vi "ReadBlueSerializableVersionPath.vi"(10 "apprefnum":u32, 11 "LVClass name":string) -> (0 "error out":errorcluster, 2 "BlueSerializableVersion found?":bool, 3 "BlueSerializableVersion":u16)   [LabVIEW 2019, in "IncrementMutationHistory.lvlib"]
uses:
  IncrementMutationHistory.lvlib
  <resource>/Framework/Providers/BlueSerializationProviderShared/UserCommentToVersion.vi
  <resource>/Framework/Providers/BlueSerializationProviderShared/BlueSerializationProviderShared.lvlib
  VILIB_NONUI/VILIB_NONUI.lvlib
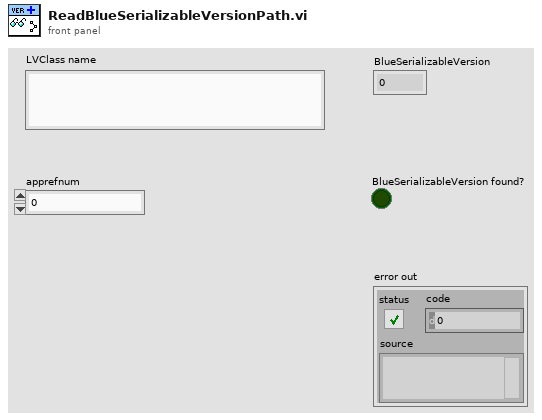
[diagram p1: front panel]
types:
  T1 = typedef "Edit LVLibs.lvlib/Mutation History.ctl" = T2[]
  T2 = typedef "Edit LVLibs.lvlib/Mutation Record.ctl" = cluster{"Library Version":T3, "Old Name Index":u8, "Class Default Data":variant, "Cluster Order Map":u32[], "Parent Name":string, "Parent Path":path, "LabVIEW Version":u32, "User Comments":string, "Mutation Flags":u8, "Parent Old Name Index":u8, "Parent Levels Added":u16, "Parent Levels Removed":u16}
  T3 = typedef "Edit LVLibs.lvlib/LibVersion.ctl" = cluster{"Major":u16, "Minor":u16, "Fix":u16, "Build":u16}
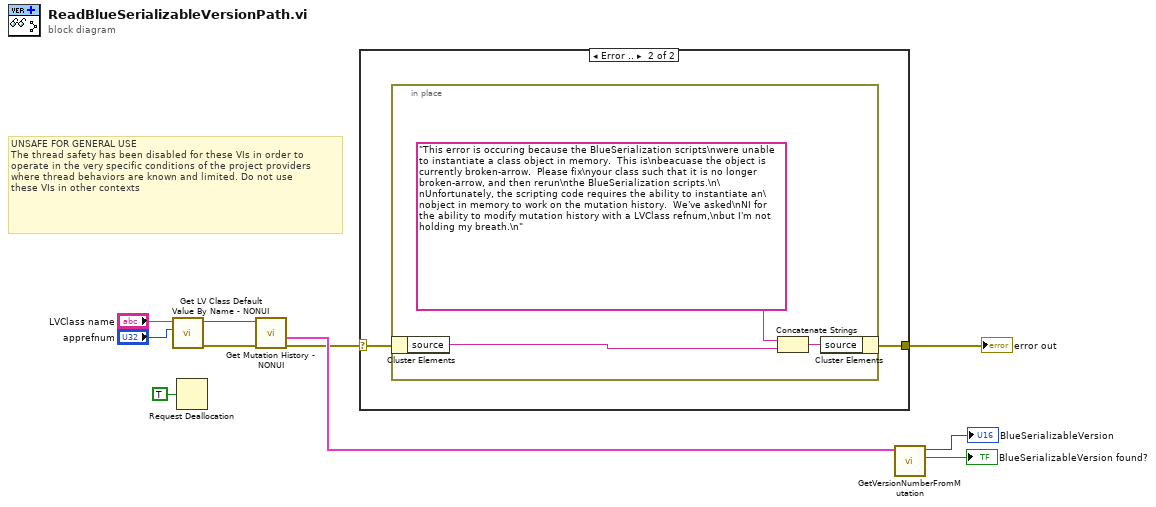
[diagram p0: block diagram]
diagram:
  # "UNSAFE FOR GENERAL USE\nThe thread safety has been disabled for these VIs in order to\noperate in the very specific conditions of the project providers\nwhere thread behaviors are known and limited. Do not use\nthese VIs in other contexts"
  n1 = call "Get LV Class Default Value By Name - NONUI.vi"("apprefnum"="apprefnum", "class name"="LVClass name") -> ("error out"=w5:errorcluster, "object"=w6:refnum<class>)  [unwired: 8 in]
  n2 = Request Deallocation(TRUE ("flag")) -> ()
  n3 = call "Get Mutation History - NONUI.vi"("error in"=w5, "Input object"=w6) -> ("error out"=w2:errorcluster, "Mutation History"=w4:T1)  [unwired: 6 in]
  n4 = case shown="Error .." w2 {
    selector: w2 -> [w11 w13]
    tunnel: [w11 w12] -> w1
    frame No Error {
    }
    frame Error {
      n5 = in-place {
        n6 = in-place-cluster #1(w13) -> ("source"=w15:string)
        n7 = Concatenate Strings("This error is occuring because the BlueSerialization scripts\nwere unable to instantiate a class object in memory.  This is\nbeacuase the object is currently broken-arrow.  Please fix\nyour class such that it is no longer broken-arrow, and then rerun\nthe BlueSerialization scripts.\n\nUnfortunately, the scripting code requires the ability to instantiate an\nobject in memory to work on the mutation history.  We've asked\nNI for the ability to modify mutation history with a LVClass refnum,\nbut I'm not holding my breath.\n", w15) -> (w14:string)
        n8 = in-place-cluster #1("source"=w14) -> (w12:errorcluster)
      }
    }
  }
  "error out" <- w1
  n9 = call <resource>:"GetVersionNumberFromMutation.vi"("Mutation History"=w4) -> ("BlueSerializableVersion found?"=→"BlueSerializableVersion found?":bool, "BlueSerializableVersion"=→"BlueSerializableVersion":u16)  [unwired: 9 in]
